vi "DynamicSubtractU8Baseline1.vi"(8 "Wrap? Input":bool, 9 "Baseline U8":u8, 10 "Trigger Edge Array":bool[](array[boolean])=[FALSE, FALSE, FALSE, FALSE], 11 "Baseline ArrayInput":u8[](array[numeric])=[0, 0, 0, 0]) -> (0 "Wrap? Output":bool, 3 "Baseline Array Output":u8[](array[numeric]))   [LabVIEW 2012]
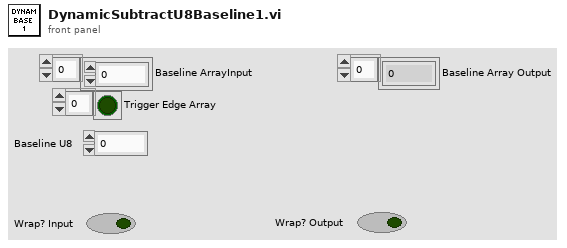
[diagram p1: front panel]
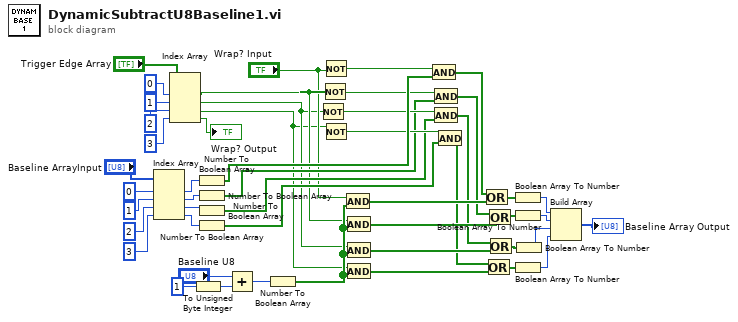
[diagram p0: block diagram]
diagram:
  n1 = Index Array(array="Baseline ArrayInput", index #1=0 ("index"), index #2=1 ("index"), index #3=2 ("index"), index #4=3 ("index")) -> (element #1=w17:u8, element #2=w16:u8, element #3=w15:u8, element #4=w14:u8)
  n2 = Index Array(array="Trigger Edge Array", index #1=0 ("index"), index #2=1 ("index"), index #3=2 ("index"), index #4=3 ("index")) -> (element #1=w3:bool, element #2=w2:bool, element #3=w1:bool, element #4=→"Wrap? Output":bool)
  n3 = To Unsigned Byte Integer(number=i16 1) -> (unsigned 8bit integer=w48:u8)
  n4 = Number To Boolean Array(number=w17) -> (Boolean array=w47:bool[])
  n5 = Number To Boolean Array(number=w16) -> (Boolean array=w11:bool[])
  n6 = Number To Boolean Array(number=w15) -> (Boolean array=w12:bool[])
  n7 = Number To Boolean Array(number=w14) -> (Boolean array=w13:bool[])
  n8 = Add(x="Baseline U8", y=w48) -> (x+y=w23:u8)
  n9 = Number To Boolean Array(number=w23) -> (Boolean array=w46:bool[])
  n10 = Not(x=w2) -> (.not. x?=w39:bool)
  n11 = Not(x=w3) -> (.not. x?=w40:bool)
  n12 = Not(x="Wrap? Input") -> (.not. x?=w41:bool)
  n13 = Not(x=w1) -> (.not. x?=w38:bool)
  n14 = And(x="Wrap? Input", y=w46) -> (x .and. y?=w29:bool[])
  n15 = And(x=w3, y=w46) -> (x .and. y?=w30:bool[])
  n16 = And(x=w2, y=w46) -> (x .and. y?=w31:bool[])
  n17 = And(x=w1, y=w46) -> (x .and. y?=w32:bool[])
  n18 = And(x=w41, y=w47) -> (x .and. y?=w28:bool[])
  n19 = And(x=w40, y=w11) -> (x .and. y?=w27:bool[])
  n20 = And(x=w39, y=w12) -> (x .and. y?=w26:bool[])
  n21 = And(x=w38, y=w13) -> (x .and. y?=w25:bool[])
  n22 = Or(x=w28, y=w29) -> (x .or. y?=w36:bool[])
  n23 = Or(x=w25, y=w32) -> (x .or. y?=w35:bool[])
  n24 = Or(x=w27, y=w30) -> (x .or. y?=w33:bool[])
  n25 = Or(x=w26, y=w31) -> (x .or. y?=w34:bool[])
  n26 = Boolean Array To Number(Boolean array=w36) -> (number=w45:u8)
  n27 = Boolean Array To Number(Boolean array=w33) -> (number=w44:u8)
  n28 = Boolean Array To Number(Boolean array=w35) -> (number=w42:u8)
  n29 = Boolean Array To Number(Boolean array=w34) -> (number=w43:u8)
  n30 = Build Array(w45, w44, w43, w42) -> (→"Baseline Array Output":u8[])
